vi "Cleanup Temp Sysdef Files.vi"(6 "bypass cleanup":bool, 8 "error in":errorcluster, 11 "Relative path":path=path "") -> (0 "error out":errorcluster)   [LabVIEW 2020, in "SLSC Switch System Tests.lvclass"]
uses:
  SLSC Switch System Tests.lvclass
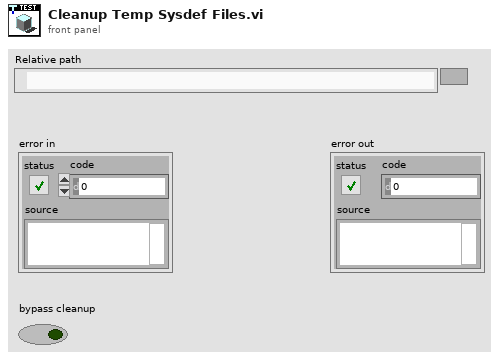
[diagram p1: front panel]
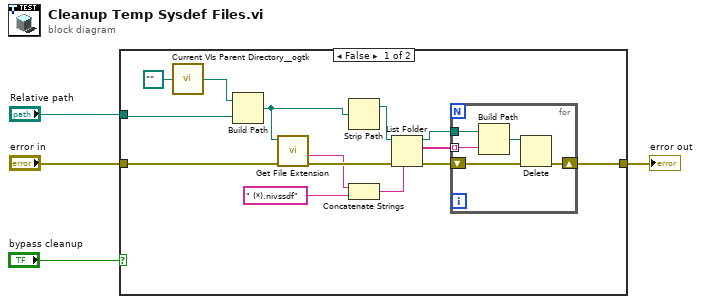
[diagram p0: block diagram]
diagram:
  n1 = case shown="False" "bypass cleanup" {
    tunnel: "Relative path" -> [w6 _]
    tunnel: "error in" -> [w14 w24]
    tunnel: [w9 w24] -> w2
    frame False {
      n2 = call <userlib>:"Current VIs Parent Directory__ogtk.vi"("Relative path (.)"=path "..") -> ("Parent Directory (+ Relative)"=w7:path)  [unwired: 4 in]
      n3 = Build Path(base path=w7, name or relative path=w6) -> (appended path=w5:path)
      n4 = call <vilib>:"Get File Extension.vi"("error in (no error)"=w14, "file"=w5) -> ("error out"=w13:errorcluster, "filename without extension"=w12:string)  [unwired: 5 in, 3 out]
      n5 = Strip Path(path=w5) -> (stripped path=w15:path)  [unwired: 1 out]
      n6 = Concatenate Strings(w12, " (*).nivssdf" ("pattern")) -> (w10:string)
      n7 = List Folder(path=w15, pattern=w10, error in=w13) -> (path out=w18:path, filenames=w17:string[], error out=w16:errorcluster)  [unwired: 1 in, 1 out]
      n8 = for {
        tunnel: w18 -> [w23]
        tunnel: w17 -> [w22] mode=indexing
        shift-right: [w19] -> w9
        shift-left: w16 -> [w20]
        n9 = Build Path(base path=w23, name or relative path=w22) -> (appended path=w21:path)
        n10 = Delete(path (use dialog)=w21, error in=w20) -> (error out=w19:errorcluster)  [unwired: 3 in, 2 out]
      }
    }
    frame True {
    }
  }
  "error out" <- w2
